vi "Read Dynamic CEID File.vi"(8 "error in (no error)":errorcluster, 11 "CEID Data In":T1[](array[typedef])) -> (0 "error out":errorcluster, 3 "CEID Data Out":T1[](array[typedef]))   [LabVIEW 2020, in "SECS Communication.lvlib" / "SECS Data Class.lvclass"]
uses:
  SECS Data Class.lvclass
  CEID Data.ctl
  PPL/Variant Parser.lvlibp
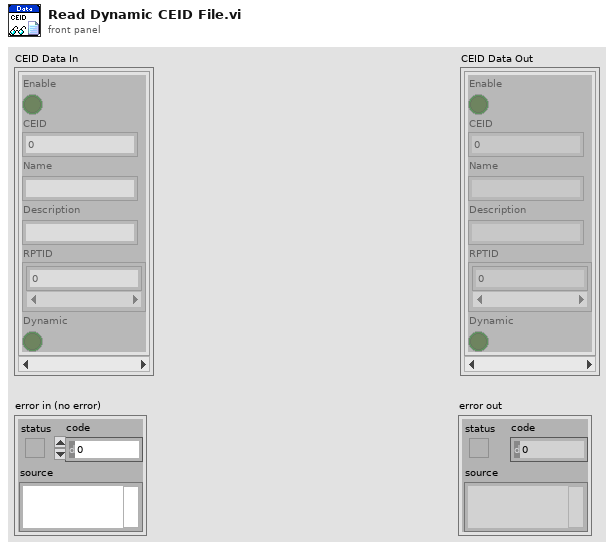
[diagram p1: front panel]
types:
  T1 = typedef "SECS Communication.lvlib/SECS Data Class.lvclass/CEID Data.ctl" = cluster{"Enable":bool, "CEID":u32, "Name":string, "Description":string, "RPTID":u32[], "Dynamic":bool}
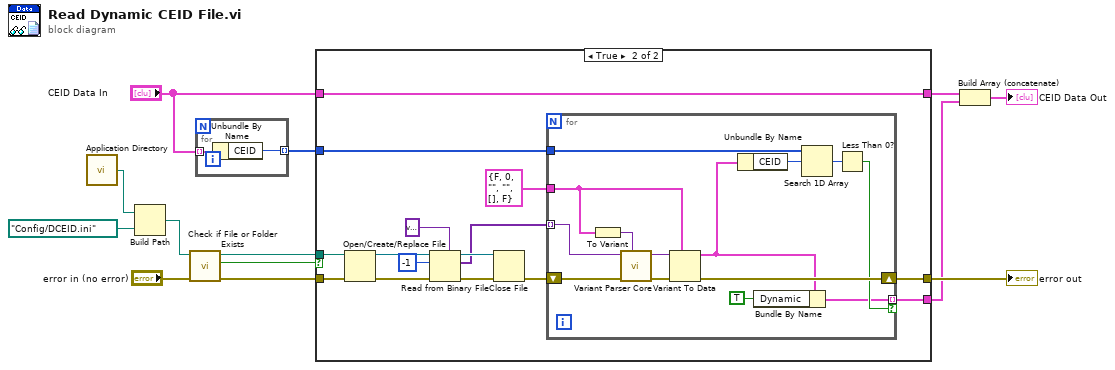
[diagram p0: block diagram]
diagram:
  n1 = call <vilib>:"Application Directory.vi"() -> ("Application Directory"=w13:path)
  n2 = Build Path(base path=w13, name or relative path=path "Config/DCEID.ini") -> (appended path=w10:path)
  n3 = call <vilib>:"Check if File or Folder Exists.vi"("error in (no error)"="error in (no error)", "path"=w10) -> ("error out"=w7:errorcluster, "file or folder exists?"=w9:bool, "dup path"=w8:path)  [unwired: 7 in]
  n4 = for {
    tunnel: "CEID Data In" -> [w15] mode=indexing
    tunnel: [w14] -> w4 mode=indexing
    n5 = Unbundle By Name(w15) -> ("CEID"=w14:u32)
  }
  n6 = case shown="True" w9 {
    tunnel: w7 -> [w17 w29]
    tunnel: w8 -> [_ w30]
    tunnel: [_ w22] -> w2
    tunnel: [w17 w21] -> w6
    tunnel: "CEID Data In" -> [w16 w19]
    tunnel: w4 -> [_ w20]
    tunnel: [w16 w19] -> w3
    frame False {
    }
    frame True {
      n7 = Open/Create/Replace File(file path (use dialog)=w30, error in=w29) -> (refnum out=w28:refnum<file>, error out=w27:errorcluster)  [unwired: 4 in, 1 out]
      n8 = Read from Binary File(5:variant, 8:w27, 10:-1 ("count (1)"), 11:w28) -> (0:w25:errorcluster, 2:w23:variant[], 3:w26:refnum<file>)  [unwired: 2 in, 1 out]
      n9 = Close File(refnum=w26, error in=w25) -> (error out=w24:errorcluster)  [unwired: 1 out]
      n10 = for {
        shift-right: [w40] -> w21
        shift-left: w24 -> [w46]
        tunnel: w23 -> [w45] mode=indexing
        tunnel: T1 {"Enable"=FALSE, "CEID"=0, "Name"="", "Description"="", "RPTID"=[], "Dynamic"=FALSE} ("CEID Data") -> [w42]
        tunnel: [w33] -> w22 mode=indexing if=w36
        tunnel: w20 -> [w39]
        n11 = To Variant(anything=w42) -> (Variant=w41:variant)
        n12 = call "Variant Parser Core.vi"("Data Type"=w41, "error in"=w46, "Variant In"=w45) -> ("error out"=w44:errorcluster, "Variant Out"=w43:variant)  [unwired: 7 in]
        n13 = Variant To Data(error in=w44, type=w42, Variant=w43) -> (data=w35:T1, error out=w40:errorcluster)
        n14 = Unbundle By Name(w35) -> ("CEID"=w38:u32)
        n15 = Bundle By Name(cluster=w35, "Dynamic"=TRUE) -> (w33:T1)
        n16 = Search 1D Array(1D array=w39, element=w38) -> (index of element=w37:i32)  [unwired: 1 in]
        n17 = Less Than 0?(x=w37) -> (x < 0?=w36:bool)
      }
    }
  }
  "error out" <- w6
  n18 = Build Array (concatenate)(w3, w2) -> (→"CEID Data Out":T1[])
